vi "Mask Write Register.vi"(4 "OR Mask":u16, 6 "AND Mask":u16, 8 "error in":errorcluster, 10 "address":u16, 11 "device data model in":refnum<class "Device Data Model.lvclass">) -> (0 "error out":errorcluster, 3 "device data model out":refnum<class "Device Data Model.lvclass">)   [LabVIEW 2021, in "Device Data Model.lvclass"]
doc: "Writes the masked value of a single register using an <b>AND mask</b> and an <b>OR mask</b> using the equation below:\nResult=(Current Value AND AndMask) OR (OrMask AND !AndMask)"
uses:
  Device Data Model.lvclass
  Device Data Model.lvclass/Device Data Model.ctl
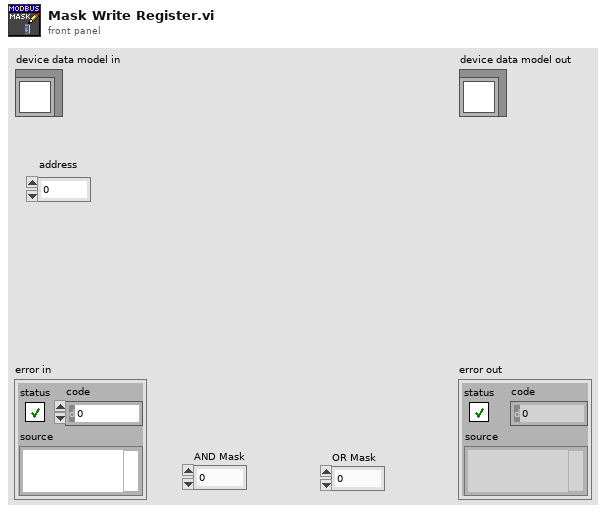
[diagram p1: front panel]
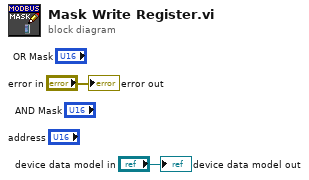
[diagram p0: block diagram]
diagram:
  "error out" <- "error in"
  "device data model out" <- "device data model in"
